vi "Pendiente_Recta.vi"() -> ()   [LabVIEW 2020]
panel:
  in  "BREAK":bool
  out "Cruce x cero":dbl
  out "Pendiente (m)":dbl
  in  "y2":dbl
  in  "y1":dbl
  in  "x2":dbl
  in  "x1":dbl
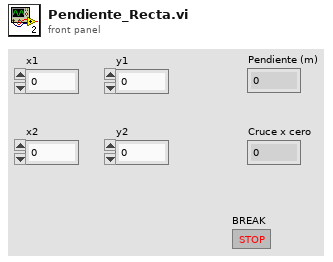
[diagram p1: front panel]
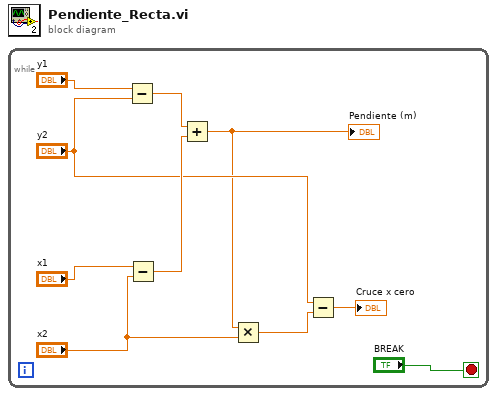
[diagram p0: block diagram]
diagram:
  n1 = while {
    stop <- "BREAK" stop-if-true
    n2 = Subtract(x="y1", y="y2") -> (x-y=w9:dbl)
    n3 = Subtract(x="x1", y="x2") -> (x-y=w8:dbl)
    n4 = Add(x=w9, y=w8) -> (x+y=w3:dbl)
    "Pendiente (m)" <- w3
    n5 = Multiply(x=w3, y="x2") -> (x*y=w4:dbl)
    n6 = Subtract(x="y2", y=w4) -> (x-y=→"Cruce x cero":dbl)
  }
